vi "Write Message Array.vi"(8 "error in (no error)":errorcluster, 10 "Message Array":refnum<class "Message.lvclass">[](array[class]), 11 "Batch Msg in":refnum<class "Batch Msg.lvclass">) -> (0 "error out":errorcluster, 3 "Batch Msg out":refnum<class "Batch Msg.lvclass">)   [LabVIEW 2020, in "Sequencer.lvlib" / "Batch Msg.lvclass"]
doc: "Write Message Array to the Batch Msg."
uses:
  Batch Msg.lvclass
  PPL/HDH.Actor Framework.Core.Actor.lvlibp/1abvi3w/vi.lib/ActorFramework/Message/Message.lvclass
  Batch Msg.lvclass/Batch Msg.ctl
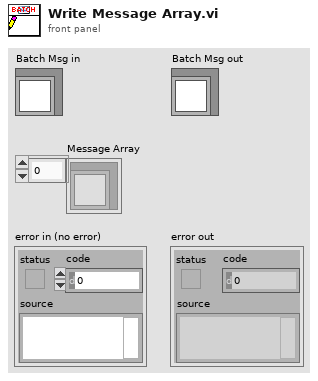
[diagram p1: front panel]
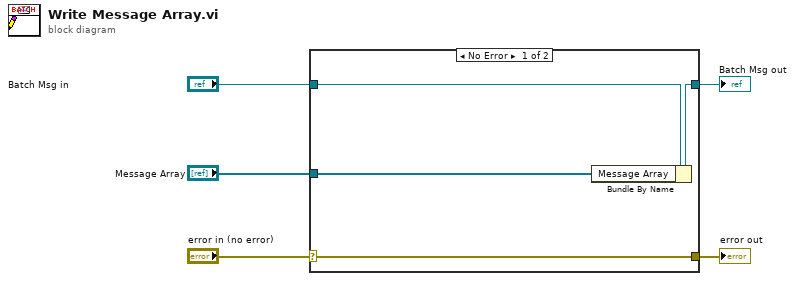
[diagram p0: block diagram]
diagram:
  n1 = case shown="No Error" "error in (no error)" {
    selector: "error in (no error)" -> [w9 w10]
    tunnel: [w9 w10] -> w4
    tunnel: [w7 w11] -> w2
    tunnel: "Batch Msg in" -> [w8 w11]
    tunnel: "Message Array" -> [w6 _]
    frame No Error {
      n2 = Bundle By Name(cluster=w8, "Message Array"=w6) -> (w7:refnum<class "Batch Msg.lvclass">)
    }
    frame Error {
    }
  }
  "error out" <- w4
  "Batch Msg out" <- w2
